vi "UpdateTraceGlobals.vi"(6 "Force Update":bool, 8 "Error In":errorcluster) -> (0 "Error Out":errorcluster)   [LabVIEW 2018, in "TracerLibrary.lvlib" / "Tracer.lvclass"]
uses:
  Tracer.lvclass
  protected/Tracer_ClassAttributes.vi
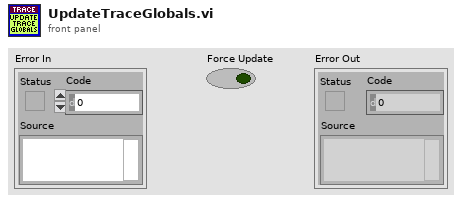
[diagram p1: front panel]
types:
  T1 = typedef "TRACE.lvlib/TRACE.lvclass/TRACE_ObjectAttributes.ctl" = cluster{"TraceContainer":variant}
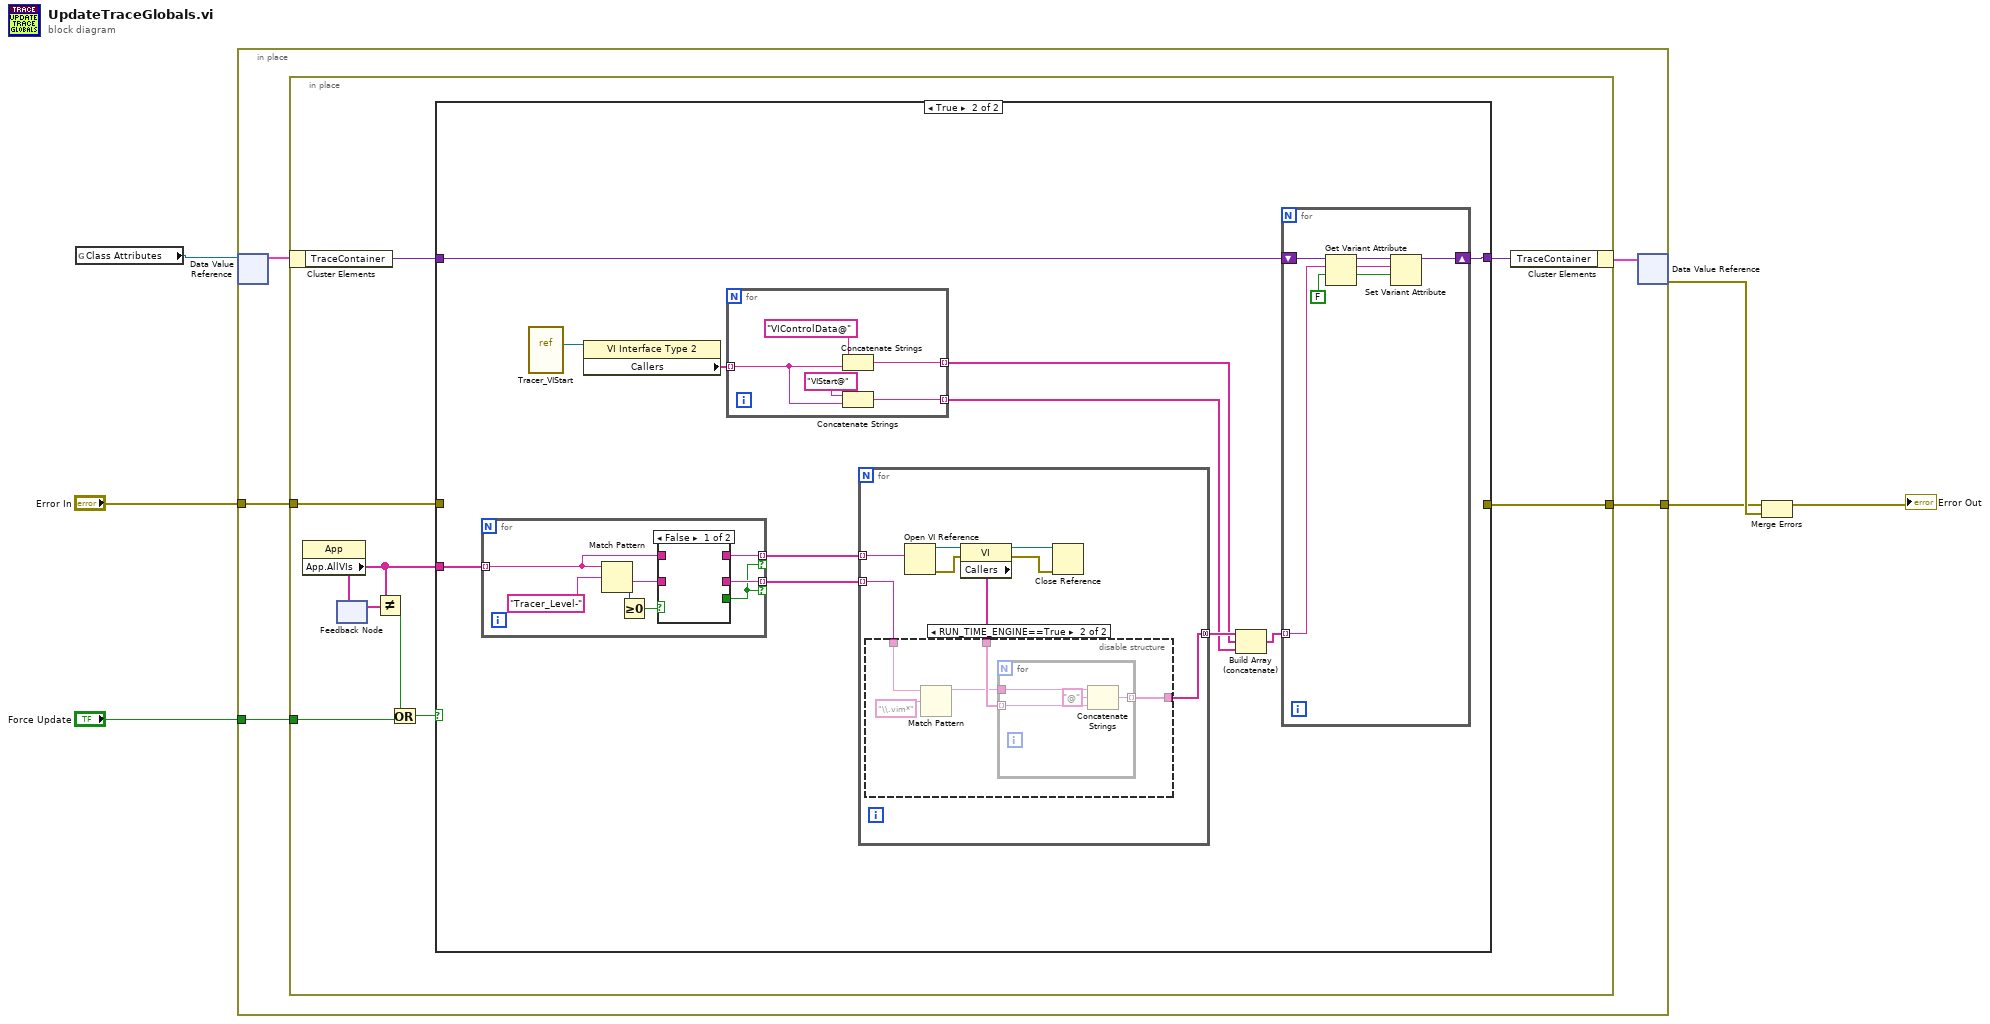
[diagram p0: block diagram]
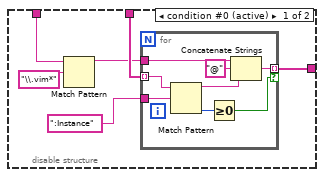
[diagram p3: hidden frame]
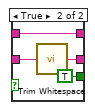
[diagram p4: hidden frame]
diagram:
  n1 = global read "Tracer_ClassAttributes.vi" "Class Attributes"() -> (w2:refnum<data-value>)
  n2 = in-place {
    in-place-border: "Error In" -> [w11]
    in-place-border: [w10] -> w3
    in-place-border: "Force Update" -> [w9]
    n3 = in-place-dvr #1(w2) -> (w8:T1)  [unwired: 1 out]
    n4 = in-place {
      in-place-border: w11 -> [w20]
      in-place-border: [w19] -> w10
      in-place-border: w9 -> [w14]
      n5 = in-place-cluster #2(w8) -> ("TraceContainer"=w13:variant)
      n6 = property class="App"() -> ("App.AllVIs"=w17:string[])  [unwired: 2 in, 2 out]
      n7 = feedback #3() -> (w18:string[])  [unwired: 1 in]
      n8 = feedback-in #3(w17) -> ()
      n9 = Not Equal?(x=w17, y=w18) -> (x != y?=w16:bool)
      n10 = Or(x=w16, y=w14) -> (x .or. y?=w15:bool)
      n11 = case shown="True" w15 {
        tunnel: w17 -> [_ w30]
        tunnel: [w21 w31] -> w12
        tunnel: w20 -> [w22 _]
        tunnel: [w22 _] -> w19
        tunnel: w13 -> [w21 w33]
        frame False {
        }
        frame True {
          n12 = for {
            tunnel: w30 -> [w76] mode=indexing
            tunnel: [w79] -> w25 mode=indexing if=w77
            tunnel: [w78] -> w26 mode=indexing if=w77
            n13 = Match Pattern(string=w76, regular expression="Tracer_Level-") -> (after substring=w80:string, offset past match=w82:i32)  [unwired: 1 in, 2 out]
            n14 = Greater Or Equal To 0?(x=w82) -> (x >= 0?=w81:bool)
            n15 = case shown="False" w81 {
              tunnel: w80 -> [_ w87]
              tunnel: [_ w86] -> w79
              tunnel: [_ TRUE] -> w77
              tunnel: [_ w84] -> w78
              tunnel: w76 -> [_ w84]
              frame False {
              }
              frame True {
                n16 = call <vilib>:"Trim Whitespace.vi"("string"=w87) -> ("trimmed string"=w86:string)  [unwired: 1 in]
              }
            }
          }
          n17 = vi-ref "Tracer_VIStart.vi"() -> (w29:refnum<vi>)
          n18 = property class="VI Interface Type 2"(reference=w29) -> ("Callers"=w24:string[])  [unwired: 1 in, 2 out]
          n19 = for {
            tunnel: w24 -> [w36] mode=indexing
            tunnel: [w37] -> w27 mode=indexing
            tunnel: [w34] -> w23 mode=indexing
            n20 = Concatenate Strings("VIControlData@" ("string"), w36) -> (w37:string)
            n21 = Concatenate Strings("VIStart@" ("string"), w36) -> (w34:string)
          }
          n22 = for {
            tunnel: w26 -> [w48] mode=indexing
            tunnel: w25 -> [w47] mode=indexing
            tunnel: [w45] -> w32 mode=concatenating
            n23 = Open VI Reference(vi path=w48) -> (vi reference=w50:refnum<vi>, error out=w52:errorcluster)  [unwired: 5 in]
            n24 = property class="VI"(reference=w50, error in=w52) -> (reference out=w49:refnum<vi>, error out=w51:errorcluster, "Callers"=w46:string[])
            n25 = disable-structure shown="RUN_TIME_ENGINE==True" {
              disable-tunnel: w47 -> [w58 w71]
              disable-tunnel: w46 -> [w57 w70]
              disable-tunnel: [w56 w69] -> w45
              frame condition #0 (active) {
                n26 = Match Pattern(string=w58, regular expression="\\.vim*") -> (before substring=w54:string)  [unwired: 1 in, 3 out]
                n27 = for {
                  tunnel: w57 -> [w63] mode=indexing
                  tunnel: w54 -> [w66]
                  tunnel: [w64] -> w56 mode=indexing if=w59
                  tunnel: ":Instance" ("regular expression") -> [w61]
                  n28 = Match Pattern(string=w63, regular expression=w61) -> (before substring=w62:string, offset past match=w60:i32)  [unwired: 1 in, 2 out]
                  n29 = Greater Or Equal To 0?(x=w60) -> (x >= 0?=w59:bool)
                  n30 = Concatenate Strings(w66, "@" ("string"), w62) -> (w64:string)
                }
              }
              frame condition #1 {
                n31 = Match Pattern(string=w71, regular expression="\\.vim*") -> (before substring=w67:string)  [unwired: 1 in, 3 out]
                n32 = for {
                  tunnel: w70 -> [w72] mode=indexing
                  tunnel: w67 -> [w75]
                  tunnel: [w73] -> w69 mode=indexing
                  n33 = Concatenate Strings(w75, "@" ("string"), w72) -> (w73:string)
                }
              }
            }
            n34 = Close Reference(reference=w49, error in (no error)=w51) -> ()  [unwired: 1 out]
          }
          n35 = Build Array (concatenate)(w32, w27, w23) -> (w28:string[])
          n36 = for {
            tunnel: w28 -> [w41] mode=indexing
            shift-right: [w39] -> w31
            shift-left: w33 -> [w44]
            n37 = Get Variant Attribute(Variant=w44, name=w41, default value (empty Variant)=FALSE) -> (duplicate Variant=w43:variant, value=w40:bool)  [unwired: 1 in, 2 out]
            n38 = Set Variant Attribute(Variant=w43, name=w41, value=w40) -> (Variant out=w39:variant)  [unwired: 1 in, 2 out]
          }
        }
      }
      n39 = in-place-cluster #2("TraceContainer"=w12) -> (w7:T1)
    }
    n40 = in-place-dvr #1(w7) -> (w6:errorcluster)  [unwired: 1 out]
  }
  n41 = Merge Errors(w3, w6) -> (→"Error Out":errorcluster)
